vi "Simulation-1 (For loop-Tunnelling)_B220061.vi"() -> ()   [LabVIEW 2021]
panel:
  out "Array":i32[](array[numeric])
  out "Numeric":i32
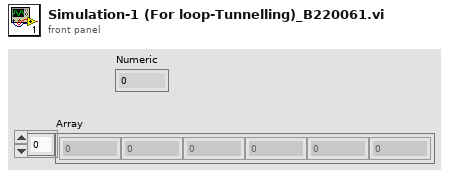
[diagram p1: front panel]
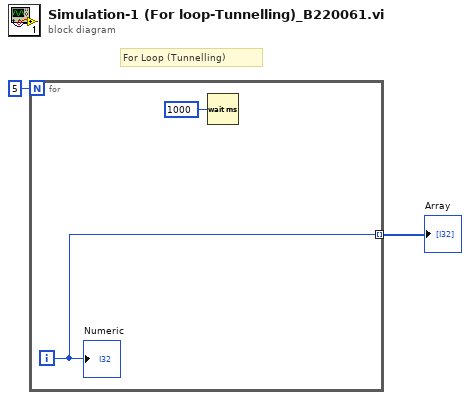
[diagram p0: block diagram]
diagram:
  # "For Loop (Tunnelling)"
  n1 = for {
    N: 5 -> [_]
    tunnel: [w3] -> w1 mode=indexing
    i -> [w3]
    n2 = Wait (ms)(milliseconds to wait=u32 1000) -> ()  [unwired: 1 out]
    "Numeric" <- w3
  }
  "Array" <- w1
